vi "VI Directory Route.vi"() -> (3 "All Folders":path[](array[path]))   [LabVIEW 2020, in "FGen.lvlib"]
uses:
  FGen.lvlib
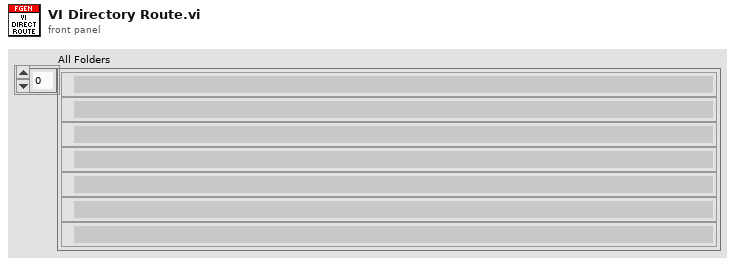
[diagram p1: front panel]
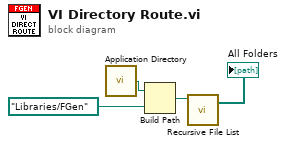
[diagram p0: block diagram]
diagram:
  n1 = call <vilib>:"Application Directory.vi"() -> ("Application Directory"=w2:path)
  n2 = Build Path(base path=w2, name or relative path=path "Libraries/FGen") -> (appended path=w4:path)
  n3 = call <vilib>:"Recursive File List.vi"("Folder Path"=w4) -> ("All Folders"=→"All Folders":path[])  [unwired: 6 in, 4 out]
